vi "print_header.vi"(8 "error in":errorcluster, 11 "inputs":T1={"path to ship file"=path "C:/Users/Lenovo/Desktop/szakdoga", "path to hand file"=path "C:/Users/Lenovo/Desktop/szakdoga", "path to gpx file"=path "C:/Users/Lenovo/Desktop/szakdoga", "hand offset"=0.0, "gps offset"=0.0, "x correction thresholds"=[], "Type"="", "Ship type"="", "Orientation"="", "Race time"="", "Other"="", "CSV Filename"=""}) -> (0 "error out":errorcluster, 3 "csv path":path)   [LabVIEW 2020]
uses:
  <vilib>/Utility/file.llb/Write Delimited Spreadsheet (string).vi
  <vilib>/regexp/Match Regular Expression.xnode
panel:
  out "x correction thresholds out":i32[](array[numeric])
  out "hand offset out":dbl
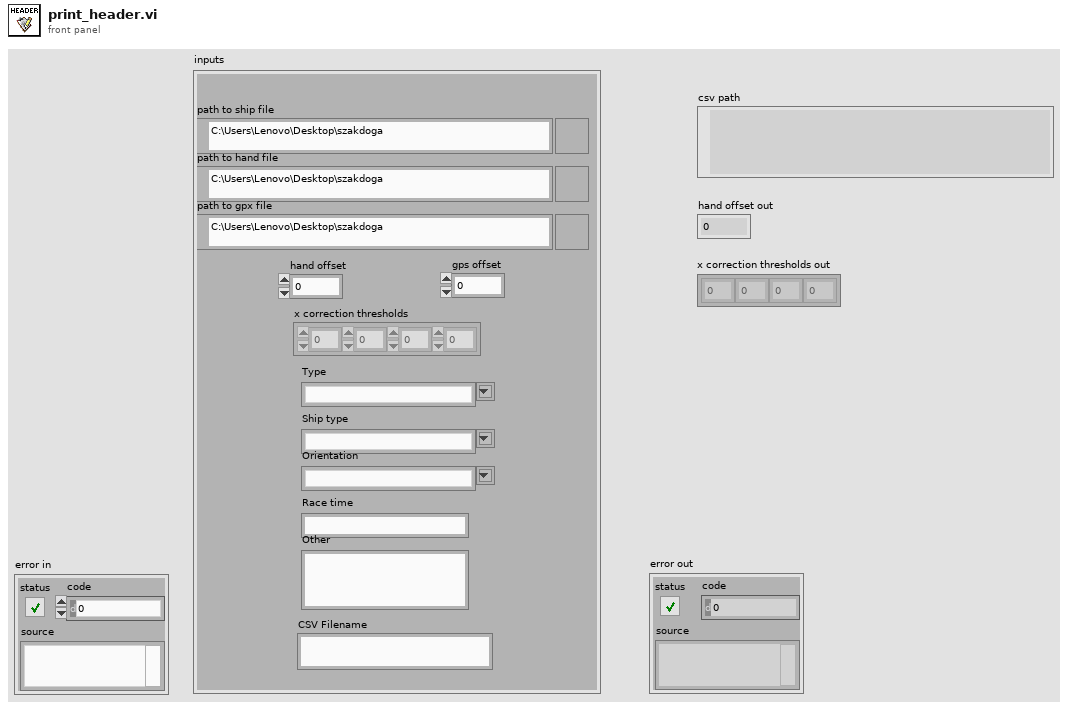
[diagram p1: front panel]
types:
  T1 = cluster{"path to ship file":path, "path to hand file":path, "path to gpx file":path, "hand offset":dbl, "gps offset":dbl, "x correction thresholds":i32[], "Type":string, "Ship type":string, "Orientation":string, "Race time":string, "Other":string, "CSV Filename":string}
  T2 = enum16{"open", "replace", "create", "open or create", "replace or create", "replace or create with confirmation"}
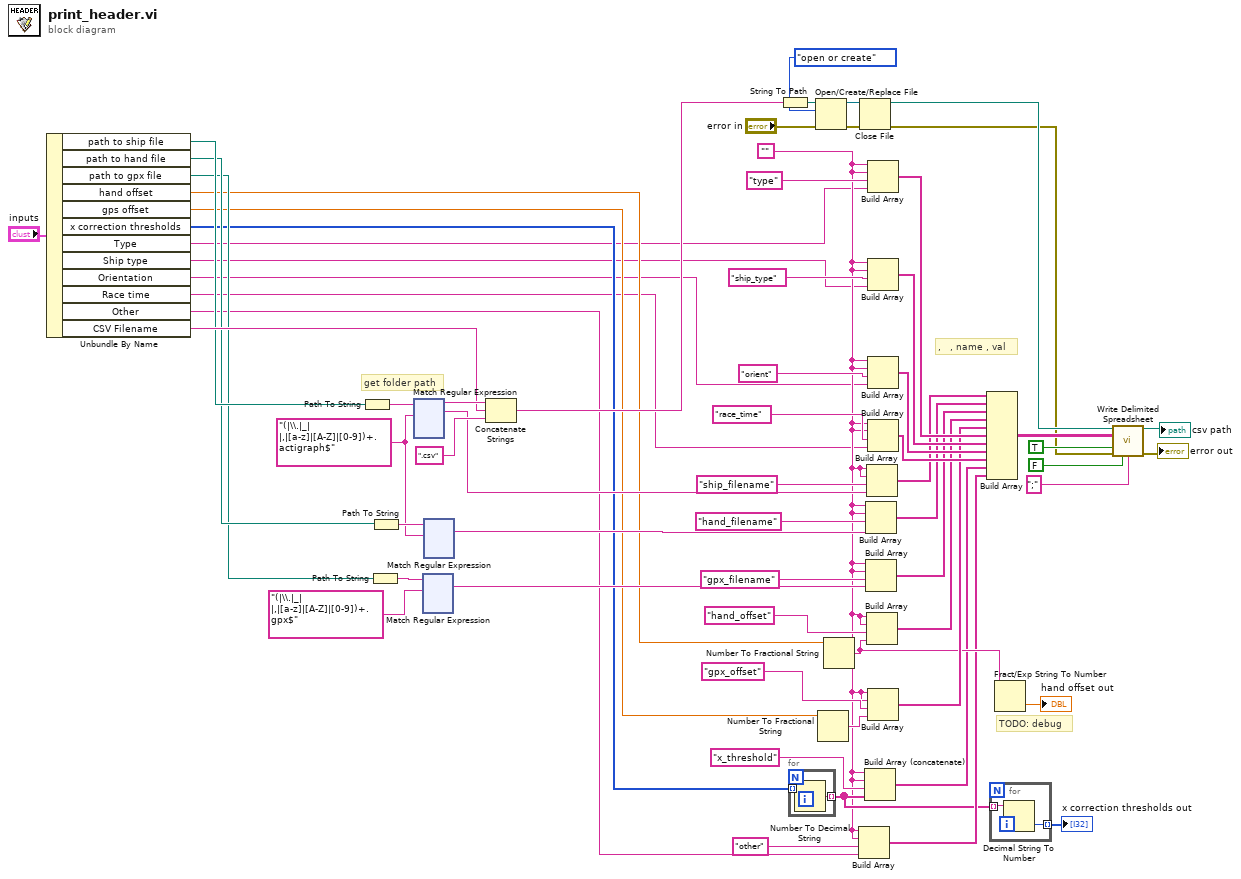
[diagram p0: block diagram]
diagram:
  w29 = "(|\\.|_| |,|[a-z]|[A-Z]|[0-9])+.actigraph$" ("regular expression")
  w11 = ""
  # "get folder path"
  # "TODO: debug"
  # ",   , name , val"
  n1 = Unbundle By Name("inputs") -> ("path to ship file"=w16:path, "path to hand file"=w15:path, "path to gpx file"=w14:path, "hand offset"=w13:dbl, "gps offset"=w12:dbl, "x correction thresholds"=w9:i32[], "Type"=w5:string, "Ship type"=w6:string, "Orientation"=w7:string, "Race time"=w8:string, "Other"=w10:string, "CSV Filename"=w17:string)
  n2 = Path To String(path=w16) -> (string=w33:string)
  n3 = Path To String(path=w14) -> (string=w31:string)
  n4 = Path To String(path=w15) -> (string=w30:string)
  n5 = xnode "Match Regular Expression"("input string"=w33, "regular expression"=w29) -> ("before match"=w34:string, "whole match"=w28:string)  [unwired: 4 in, 3 out]
  n6 = xnode "Match Regular Expression"("input string"=w31, "regular expression"="(|\\.|_| |,|[a-z]|[A-Z]|[0-9])+.gpx$") -> ("whole match"=w26:string)  [unwired: 4 in, 4 out]
  n7 = xnode "Match Regular Expression"("input string"=w30, "regular expression"=w29) -> ("whole match"=w27:string)  [unwired: 4 in, 4 out]
  n8 = Concatenate Strings(w34, w17, ".csv" ("extension")) -> (w19:string)
  n9 = String To Path(string=w19) -> (path=w24:path)
  n10 = for {
    tunnel: w9 -> [w67] mode=indexing
    tunnel: [w66] -> w36 mode=indexing
    n11 = Number To Decimal String(number=w67) -> (decimal integer string=w66:string)  [unwired: 1 in]
  }
  n12 = Open/Create/Replace File(file path (use dialog)=w24, error in="error in", operation (0:open)=T2."open or create") -> (refnum out=w22:refnum<file>, error out=w23:errorcluster)  [unwired: 3 in, 1 out]
  n13 = Number To Fractional String(number=w12) -> (F-format string=w43:string)  [unwired: 3 in]
  n14 = Number To Fractional String(number=w13) -> (F-format string=w45:string)  [unwired: 3 in]
  n15 = Build Array(w11, w11, "other", w10) -> (w37:string[])
  n16 = Close File(refnum=w22, error in=w23) -> (path=w21:path, error out=w20:errorcluster)
  n17 = Build Array (concatenate)(w11, w11, "x_threshold", w36) -> (w38:string[])
  n18 = Build Array(w11, w11, "hand_filename", w27) -> (w50:string[])
  n19 = Build Array(w11, w11, "gpx_filename", w26) -> (w49:string[])
  n20 = Build Array(w11, w11, "ship_filename", w28) -> (w40:string[])
  n21 = Build Array(w11, w11, "hand_offset", w45) -> (w47:string[])
  n22 = Build Array(w11, w11, "type", w5) -> (w59:string[])
  n23 = Build Array(w11, w11, "ship_type", w6) -> (w58:string[])
  n24 = Build Array(w11, w11, "orient", w7) -> (w55:string[])
  n25 = Build Array(w11, w11, "race_time", w8) -> (w54:string[])
  n26 = Build Array(w11, w11, "gpx_offset", w43) -> (w46:string[])
  n27 = Build Array(w40, w50, w49, w47, w46, w59, w58, w55, w54, w38, w37) -> (w62:string[][])
  n28 = for {
    tunnel: w36 -> [w69] mode=indexing
    tunnel: [w68] -> w35 mode=indexing
    n29 = Decimal String To Number(string=w69) -> (number=w68:i32)  [unwired: 2 in, 1 out]
  }
  "x correction thresholds out" <- w35
  n30 = Fract/Exp String To Number(string=w45) -> (number=→"hand offset out":dbl)  [unwired: 3 in, 1 out]
  n31 = call-poly <vilib>:"Write Delimited Spreadsheet.vi"("file path (dialog if empty)"=w21, "2D data"=w62, "append to file? (new file:F)"=TRUE, "error in (no error)"=w20, "transpose? (no:F)"=FALSE, "delimiter (\\t)"=";" ("element")) -> ("new file path (Not A Path if cancelled)"=→"csv path":path, "error out"=→"error out":errorcluster)  [unwired: 8 in]
